vi "write single param.vi"(8 "error in (no error)":errorcluster, 10 "string":string, 11 "PSP-603 in":refnum<class "PSP-603.lvclass">) -> (0 "error out":errorcluster, 3 "PSP-603 out":refnum<class "PSP-603.lvclass">)   [LabVIEW 2025, in "Power Supply.lvlib" / "PSP-603.lvclass"]
uses:
  PSP-603.lvclass
  PSP-603.lvclass/PSP-603.ctl
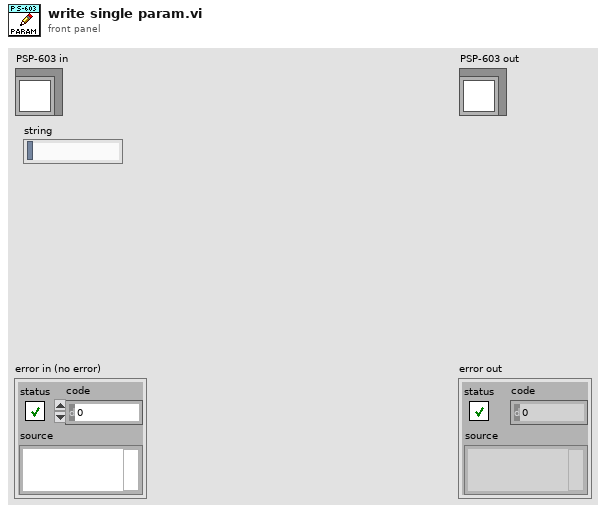
[diagram p1: front panel]
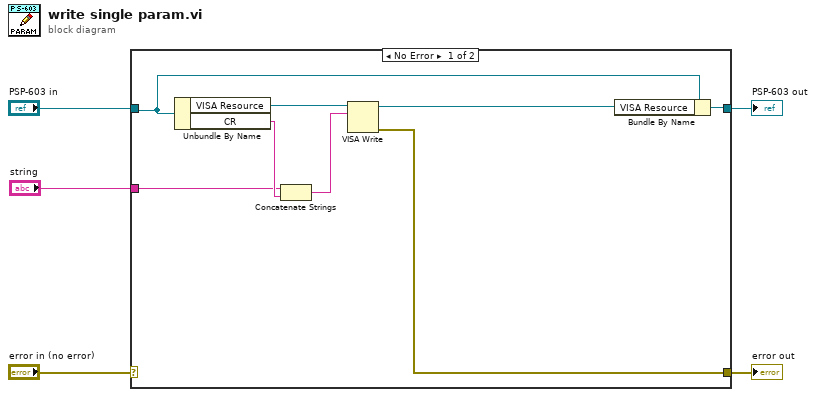
[diagram p0: block diagram]
diagram:
  n1 = case shown="No Error" "error in (no error)" {
    selector: "error in (no error)" -> [_ w15]
    tunnel: [w6 w15] -> w4
    tunnel: [w12 w14] -> w2
    tunnel: "PSP-603 in" -> [w11 w14]
    tunnel: "string" -> [w8 _]
    frame No Error {
      n2 = Unbundle By Name(w11) -> ("VISA Resource"=w13:refnum<visa-resource-name>, "CR"=w9:string)
      n3 = Concatenate Strings(w8, w9) -> (w7:string)
      n4 = VISA Write(VISA resource name=w13, write buffer=w7) -> (VISA resource name out=w10:refnum<visa-resource-name>, error out=w6:errorcluster)  [unwired: 1 in, 1 out]
      n5 = Bundle By Name(cluster=w11, "VISA Resource"=w10) -> (w12:refnum<class "PSP-603.lvclass">)
    }
    frame Error {
    }
  }
  "error out" <- w4
  "PSP-603 out" <- w2
